vi "Shutdown.vi"(8 "error in (no error)":errorcluster, 11 "TCP Client in":refnum<class "TCP Client.lvclass">) -> (0 "error out":errorcluster, 3 "TCP Client out":refnum<class "TCP Client.lvclass">)   [LabVIEW 2020, in "Stream-TCP.lvlib" / "TCP Client.lvclass"]
uses:
  TCP Client.lvclass
  Client Command.ctl
  Connection State.ctl
  TCP Client.lvclass/TCP Client.ctl
  Stream-TCP.lvlib
  lv-trace/Trace/Trace.lvlib
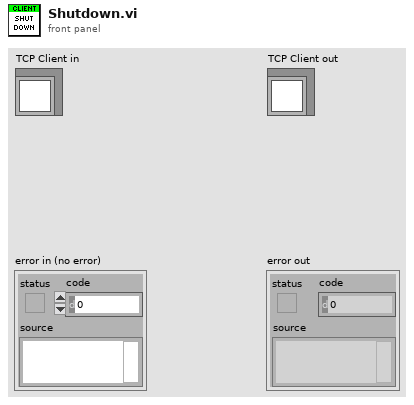
[diagram p1: front panel]
types:
  T1 = typedef "Stream-TCP.lvlib/TCP Client.lvclass/Connection State.ctl" = enum16{"Closed", "Idle", "Connecting", "Connected", "Shutdown"}
  T2 = typedef "Stream-TCP.lvlib/Client Command.ctl" = enum16{"Connect", "Close", "Shutdown", "Reconnect"}
  T3 = typedef "Stream-TCP.lvlib/Client Command Queue.ctl" = refnum<queue>
  T4 = typedef "Stream-TCP.lvlib/TCP Client.lvclass/Ref Data.ctl" = cluster{"TCP Connection":refnum<k5>, "TCP Stream":refnum<class "TCP Stream.lvclass">, "State":T1, "Connection Loop":refnum<vi>, "TCP Mode":T5, "Timeout ms":i32, "Server Connection":bool}
  T5 = typedef "Stream-TCP.lvlib/TCP Mode.ctl" = enum16{"buffered", "raw"}
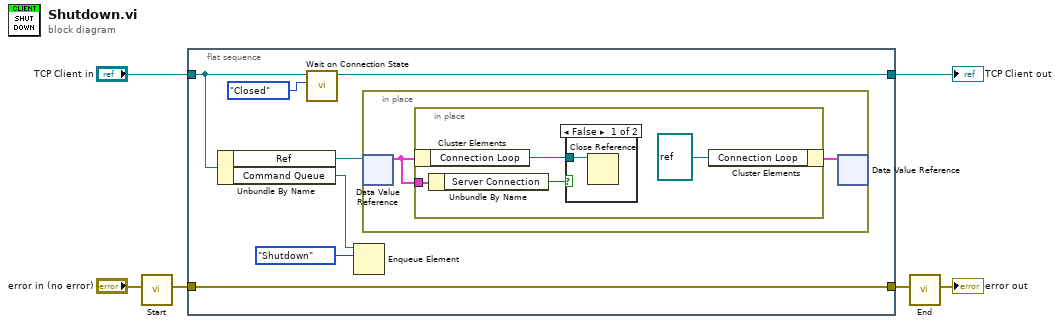
[diagram p0: block diagram]
diagram:
  n1 = call "Start.vi"("error in (no error)"="error in (no error)") -> ("error out"=w3:errorcluster)  [unwired: 10 in]
  n2 = flat-sequence {
    tunnel: "TCP Client in" -> [w11]
    tunnel: [w9] -> w5
    tunnel: w3 -> [w8]
    tunnel: [w8] -> w2
    frame #0 {
      n3 = Unbundle By Name(w11) -> ("Ref"=w7:refnum<data-value>, "Command Queue"=w13:T3)
      n4 = call "Wait on Connection State.vi"("Connection State"=Connection_State."Closed", "TCP Client in"=w11) -> ("TCP Client out"=w9:refnum<class "TCP Client.lvclass">)  [unwired: 7 in, 2 out]
      n5 = Enqueue Element(queue=w13, element=Client_Command."Shutdown") -> ()  [unwired: 2 in, 3 out]
      n6 = in-place {
        n7 = in-place-dvr #1(w7) -> (w14:T4)  [unwired: 1 out]
        n8 = in-place {
          in-place-border: w14 -> [w17]
          n9 = in-place-cluster #2(w14) -> ("Connection Loop"=w18:refnum<vi>)
          n10 = Unbundle By Name(w17) -> ("Server Connection"=w16:bool)
          n11 = case shown="False" w16 {
            tunnel: w18 -> [w20 _]
            frame False {
              n12 = Close Reference(reference=w20) -> ()  [unwired: 1 in, 1 out]
            }
            frame True {
            }
          }
          n13 = in-place-cluster #2("Connection Loop"=refnum<vi> refnum) -> (w15:T4)
        }
        n14 = in-place-dvr #1(w15) -> ()  [unwired: 2 out]
      }
    }
  }
  n15 = call "End.vi"("error in (no error)"=w2) -> ("error out"=→"error out":errorcluster)  [unwired: 10 in]
  "TCP Client out" <- w5
